vi "path.vi"() -> ()   [LabVIEW 2016]
uses:
  <vilib>/imath/engines/lvmath2/RunTimeEngine/NodeEndStatement/NIMS_NodeEndStatement_Output.vi
  <instcachedir>/0/NIMS_NodeEndStatement_Output_53EC0D466D134D7ABD903AC30B43404B.lvgen/NIMS_NodeEndStatement_Output_53EC0D466D134D7ABD903AC30B43404B_011.vi
  <vilib>/imath/engines/lvmath2/RunTimeEngine/ErrorHandling/NIMS_Finalize Error.vi
  <vilib>/imath/engines/lvmath2/RunTimeEngine/IndexRead/NIMS M($,S).vi
  <instcachedir>/0/NIMS M($,S)_3E5749BBB62E49528D4765A77F1F6D98.lvgen/NIMS M($,S)_3E5749BBB62E49528D4765A77F1F6D98_000.vi
  <vilib>/imath/engines/lvmath2/RunTimeEngine/ArithmeticOperatorToken/NIMS_ArithmeticOperator_minus.vi
  <instcachedir>/0/NIMS_ArithmeticOperator_minus_E3B65B1D26A44BB184AFDC5B3F458E3D.lvgen/NIMS_ArithmeticOperator_minus_E3B65B1D26A44BB184AFDC5B3F458E3D_017.vi
  <vilib>/imath/engines/lvmath2/RunTimeEngine/BuiltInFunctions/norm/NIMS_norm(GV,DBL).vi
  <instcachedir>/0/NIMS_norm(GV,DBL)_1268AFF3C646412B8C6EA3CE75D09042.lvgen/NIMS_norm(GV,DBL)_1268AFF3C646412B8C6EA3CE75D09042_000.vi
  <vilib>/imath/engines/lvmath2/RunTimeEngine/ErrorHandling/NIMS_Create Error From Enums.vi
  <vilib>/imath/engines/lvmath2/RunTimeEngine/IndexRead/NIMS M($,R2).vi
  <instcachedir>/0/NIMS M($,R2)_D9380E19261A4ADFB2D364AF6959C6EF.lvgen/NIMS M($,R2)_D9380E19261A4ADFB2D364AF6959C6EF_001.vi
  <vilib>/imath/engines/lvmath2/RunTimeEngine/RowToken/NIMS_RowToken_M_CV.vi
  <instcachedir>/0/NIMS_RowToken_M_CV_FA79F1D1D17D44459F3ED8E09EE8B625.lvgen/NIMS_RowToken_M_CV_FA79F1D1D17D44459F3ED8E09EE8B625_000.vi
  <vilib>/imath/engines/lvmath2/RunTimeEngine/BuiltInFunctions/size/NIMS_I32=size(GM,I32).vi
  <instcachedir>/0/NIMS_I32=size(GM,I32)_122058B1B3294FAEA5DC209B92B394E4.lvgen/NIMS_I32=size(GM,I32)_122058B1B3294FAEA5DC209B92B394E4_004.vi
  <vilib>/imathl/engines/lvmath/Functions/Error Handling/Create Error.vi
  <vilib>/imath/engines/lvmath2/RunTimeEngine/RangeToken/NIMS_Range_R2 - Integer.vi
  <instcachedir>/0/NIMS_Range_R2 - Integer_89B873E74E6E489885E44F751DD9C6BF.lvgen/NIMS_Range_R2 - Integer_89B873E74E6E489885E44F751DD9C6BF_000.vi
  <vilib>/imath/engines/lvmath2/RunTimeEngine/CommandStatement/MC_CommandStatement_break.vi
  <instcachedir>/0/NIMS_ArithmeticOperator_minus_E3B65B1D26A44BB184AFDC5B3F458E3D.lvgen/NIMS_ArithmeticOperator_minus_E3B65B1D26A44BB184AFDC5B3F458E3D_003.vi
  <vilib>/imath/engines/lvmath2/RunTimeEngine/VariableToken/NIMS_VariableToken_CondDefined.vi
  <instcachedir>/0/NIMS_VariableToken_CondDefined_06E9DA95BD4D46A6BA55EC651A891960.lvgen/NIMS_VariableToken_CondDefined_06E9DA95BD4D46A6BA55EC651A891960_009.vi
  <vilib>/imath/engines/lvmath/Functions/Error Handling/MergeErrorsWrapper.vi
  <instcachedir>/0/NIMS_NodeEndStatement_Output_53EC0D466D134D7ABD903AC30B43404B.lvgen/NIMS_NodeEndStatement_Output_53EC0D466D134D7ABD903AC30B43404B_005.vi
  <instcachedir>/0/NIMS_NodeEndStatement_Output_53EC0D466D134D7ABD903AC30B43404B.lvgen/NIMS_NodeEndStatement_Output_53EC0D466D134D7ABD903AC30B43404B_010.vi
  <vilib>/imath/engines/lvmath2/RunTimeEngine/BuiltInFunctions/length/NIMS_length(GM).vi
  <instcachedir>/0/NIMS_length(GM)_47CEC356FCE0482D9BA47DC61C99F2C7.lvgen/NIMS_length(GM)_47CEC356FCE0482D9BA47DC61C99F2C7_000.vi
  <instcachedir>/0/NIMS_ArithmeticOperator_minus_E3B65B1D26A44BB184AFDC5B3F458E3D.lvgen/NIMS_ArithmeticOperator_minus_E3B65B1D26A44BB184AFDC5B3F458E3D_012.vi
  <vilib>/imath/engines/lvmath2/RunTimeEngine/IndexRead/NIMS V(S).vi
  <instcachedir>/0/NIMS V(S)_0488751826AF41519A22953C041130DC.lvgen/NIMS V(S)_0488751826AF41519A22953C041130DC_000.vi
  <instcachedir>/0/NIMS V(S)_0488751826AF41519A22953C041130DC.lvgen/NIMS V(S)_0488751826AF41519A22953C041130DC_002.vi
  <vilib>/imath/engines/lvmath2/RunTimeEngine/BuiltInFunctions/dot/NIMS_dot(GV,GV).vi
  <instcachedir>/0/NIMS_dot(GV,GV)_B9FAA411F4494E9B94D442721014A3FA.lvgen/NIMS_dot(GV,GV)_B9FAA411F4494E9B94D442721014A3FA_000.vi
  <instcachedir>/0/NIMS_NodeEndStatement_Output_53EC0D466D134D7ABD903AC30B43404B.lvgen/NIMS_NodeEndStatement_Output_53EC0D466D134D7ABD903AC30B43404B_009.vi
panel:
  out "添加的数组 2":sgl[](array[numeric])
  out "队列中元素数量 2":i32
  out "添加的数组":sgl[](array[numeric])
  out "speed_send":dbl[](array[numeric])
  out "vertices_send":dbl[](array[numeric])
  out "angle_send":dbl[](array[numeric])
  out "路径规划数据写入缓冲区":string
  in  "目标位置3":dbl[](array[numeric])=[2645.0, 2645.0]
  in  "目标位置2":dbl[](array[numeric])=[6000.0, 1500.0]
  in  "目标位置1":dbl[](array[numeric])=[9355.0, 2645.0]
  in  "初始位置":dbl[](array[numeric])=[12000.0, 0.0]
  in  "Key2(点3)":bool
  in  "Key1(点2)":bool
  in  "Key0(点1)":bool
  out "队列中元素数量":i32
  in  "speed_max":dbl=3000.0
  in  "发送写入":refnum<visa-resource-name>
  in  "全场定位串口":refnum<visa-resource-name>="ASRL6::INSTR"
  in  "串口设置（全场定位）":T1={"波特率"=115200, "数据位"=8, "校验"=enum."None", "停止位"=10, "流控制"=0} {"流控制" items=["无"=0, "XON/XOFF"=1, "RTS/CTS"=2, "DTR/DSR"=4]; "停止位" items=["1.0"=10, "1.5"=15, "2.0"=20]; "数据位" min=5 max=8 step=1; "波特率" items=["115200"=115200, "460800"=460800, "75"=75, "110"=110, "134"=134, "150"=150, "300"=300, "600"=600, "1200"=1200, "1800"=1800, "2400"=2400, "4800"=4800, "7200"=7200, "9600"=9600, "14400"=14400, "19200"=19200, "28800"=28800, "38400"=38400, "56000"=56000, "57600"=57600, "128000"=128000, "230400"=230400]}
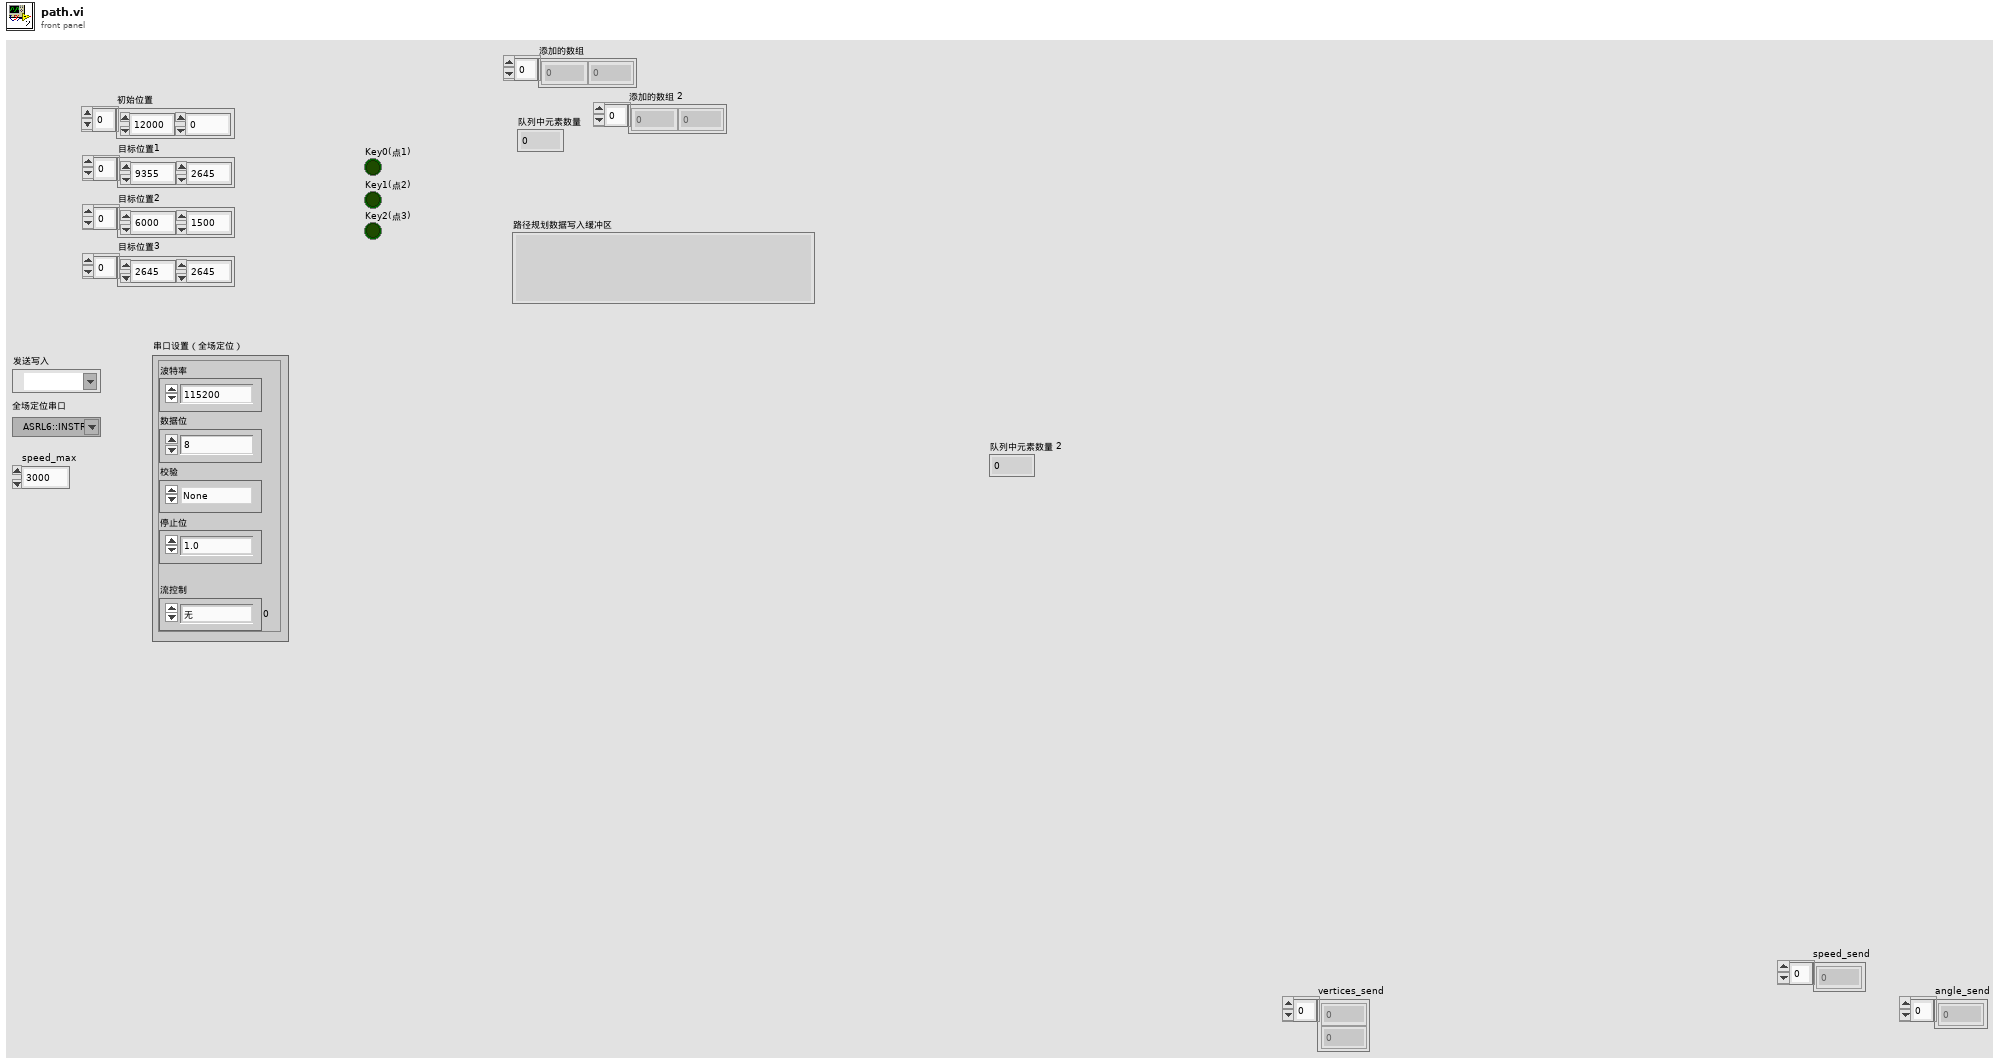
[diagram p1: front panel]
types:
  T1 = cluster{"波特率":u32, "数据位":u16, "校验":enum16{"None", "Odd", "Even", "Mark", "Space"}, "停止位":u16, "流控制":u16}
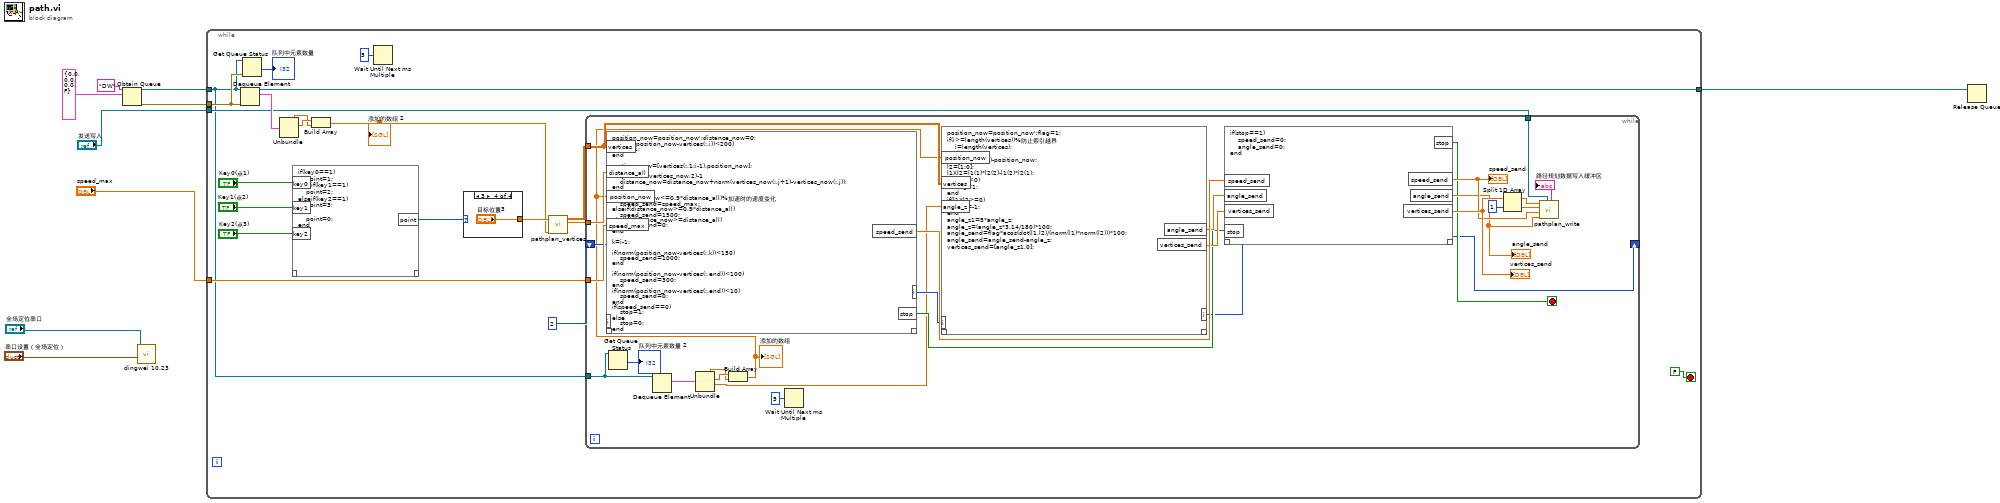
[diagram p0: block diagram]
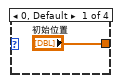
[diagram p2: hidden frame]
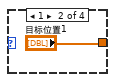
[diagram p3: hidden frame]
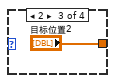
[diagram p4: hidden frame]
diagram:
  n1 = Obtain Queue(name (unnamed)="DW" ("名称（未命名）"), element data type=cluster{sgl, sgl, sgl, bool} {0.0, 0.0, 0.0, FALSE} ("输出簇 2")) -> (queue out=w5:refnum<queue>, error out=w4:errorcluster)  [unwired: 3 in, 1 out]
  n2 = call "dingwei 10.23.vi"("串口设置（遥控器）"="串口设置（全场定位）", "VISA resource name"="全场定位串口") -> ()  [unwired: 10 in]
  n3 = while {
    tunnel: w5 -> [w12]
    tunnel: w4 -> [w28]
    tunnel: [w13] -> w3
    tunnel: "speed_max" -> [w17]
    tunnel: "发送写入" -> [w14]
    stop <- FALSE stop-if-true
    n4 = Dequeue Element(queue=w12, error in (no error)=w28) -> (queue out=w13:refnum<queue>, element=w27:cluster{sgl, sgl, sgl, bool})  [unwired: 1 in, 2 out]
    n5 = Get Queue Status(queue=w12, error in (no error)=w28) -> (# elements in queue=→"队列中元素数量":i32)  [unwired: 1 in, 7 out]
    n6 = Unbundle(w27) -> (w10:sgl, w11:sgl)  [unwired: 2 out]
    n7 = mathscript code="if(key0==1)\n    point=1;\nelseif(key1==1)\n    point=2;\nelseif(key2==1)\n    point=3;\nelse\n    point=0;\nend"("key0"="Key0(点1)", "key1"="Key1(点2)", "key2"="Key2(点3)") -> ("point"=w22:i32)  [unwired: 1 in, 1 out]
    n8 = Build Array(w11, w10) -> (w16:sgl[])
    "添加的数组 2" <- w16
    n9 = Wait Until Next ms Multiple(millisecond multiple=u32 5 ("等待时间（毫秒）")) -> ()  [unwired: 1 out]
    n10 = case shown="3" w22 {
      tunnel: ["初始位置" "目标位置1" "目标位置2" "目标位置3"] -> w21
      frame 0, Default {
      }
      frame 1 {
      }
      frame 2 {
      }
      frame 3 {
      }
    }
    n11 = call "pathplan_vertices.vi"("终点"=w21, "起点"=w16) -> ("vertices"=w18:dbl[][], "distance_all"=w19:dbl)  [unwired: 5 in, 2 out]
    n12 = while {
      tunnel: w19 -> [w48]
      tunnel: w18 -> [w46]
      tunnel: w17 -> [w47]
      shift-right: [w39] -> _
      shift-left: 2 -> [w41]
      tunnel: w14 -> [w38]
      tunnel: w12 -> [w34]
      stop <- w49 stop-if-true
      n13 = Get Queue Status(queue=w34) -> (# elements in queue=→"队列中元素数量 2":i32)  [unwired: 2 in, 7 out]
      n14 = Dequeue Element(queue=w34) -> (element=w37:cluster{sgl, sgl, sgl, bool})  [unwired: 2 in, 3 out]
      n15 = Unbundle(w37) -> (w31:sgl, w32:sgl, w30:sgl)  [unwired: 1 out]
      n16 = Build Array(w32, w31) -> (w36:sgl[])
      "添加的数组" <- w36
      n17 = mathscript code="position_now=position_now';distance_now=0;\nif(norm(position_now-vertices(:,i))<200)\n    i=i+1;\nend\n\nvertices_now=[vertices(:,1:i-1),position_now];\n\nfor j=1:size(vertices_now,2)-1\n    distance_now=distance_now+norm(vertices_now(:,j+1)-vertices_now(:,j));\nend\n\nif(distance_now<=0.9*distance_all)%加速时的速度变化\n    speed_send=speed_max;\nelseif(distance_now>=0.9*distance_all)\n    speed_send=1500;\nelseif(distance_now>=distance_all)\n    speed_send=0;\nend\n\nk=i-1;\n\nif(norm(position_now-vertices(:,k))<150)\n    speed_send=1000;\nend\n\nif(norm(position_now-vertices(:,end))<100)\n    speed_send=300;\nend\nif(norm(position_now-vertices(:,end))<10)\n    speed_send=0;\nend\nif(speed_send==0)\n    stop=1;\nelse\n    stop=0;\nend"("position_now"=w36, "vertices"=w46, "distance_all"=w48, "i"=w41, "speed_max"=w47) -> ("i"=w40:i32, "speed_send"=w45:dbl[], "stop"=w42:bool)  [unwired: 1 in, 1 out]
      n18 = Wait Until Next ms Multiple(millisecond multiple=u32 5 ("毫秒倍数")) -> ()  [unwired: 1 out]
      n19 = mathscript code="position_now=position_now';flag=1;\nif(i>=length(vertices))%防止索引越界\n    i=length(vertices);\nend\nl1=vertices(:,i)-position_now;\nl2=[1;0];\nl1Xl2=l1(1)*l2(2)-l1(2)*l2(1);\nif(l1Xl2<0)\n    flag=1;\nend\nif(l1Xl2>=0)\n    flag=-1;\nend\nangle_z1=5*angle_z;\nangle_z=(angle_z*3.14/180)*100;\nangle_send=flag*acos(dot(l1,l2)/(norm(l1)*norm(l2)))*100;\nangle_send=angle_send-angle_z;\nvertices_send=[angle_z1,0];"("position_now"=w36, "angle_z"=w30, "i"=w40, "vertices"=w46) -> ("i"=w39:i32, "angle_send"=w44:cdb, "vertices_send"=w43:dbl[])  [unwired: 1 in, 1 out]
      n20 = mathscript code="if(stop==1)\n    speed_send=0;\n    angle_send=0;\nend"("speed_send"=w45, "angle_send"=w44, "vertices_send"=w43, "stop"=w42) -> ("angle_send"=w51:dbl[], "speed_send"=w52:dbl[], "vertices_send"=w53:dbl[], "stop"=w49:bool)  [unwired: 1 in, 1 out]
      "speed_send" <- w52
      "vertices_send" <- w53
      "angle_send" <- w51
      n21 = Split 1D Array(array=w53, index=1 ("索引")) -> (first subarray=w55:dbl[], second subarray=w54:dbl[])
      n22 = call "pathplan_write.vi"("VISA资源名称"=w38, "angle"=w51, "v"=w52, "y"=w54, "angle_err"=w55) -> ("路径规划数据写入缓冲区"=→"路径规划数据写入缓冲区":string)  [unwired: 6 in]
    }
  }
  n23 = Release Queue(queue=w3) -> ()  [unwired: 2 in, 3 out]
